vi "DB_EscribeTablaEventos.vi"(8 "error in (no error)":errorcluster, 11 "DESCRIPCION":string) -> (0 "error out":errorcluster)   [LabVIEW 2018]
uses:
  <vilib>/addons/database/Connection.llb/DB Tools Open Connec (Path).vi
  <vilib>/addons/database/Connection.llb/Conn Execute.vi
  <vilib>/addons/database/Recordset.llb/Rec Destroy - Connection.vi
  <vilib>/addons/database/NI_Database_API.lvlib
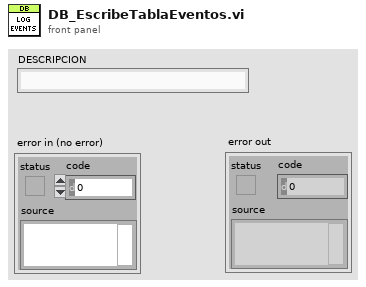
[diagram p1: front panel]
types:
  T1 = typedef "NI_Database_API.lvlib/Conn ObjectReference.ctl" = refnum<k1>
  T2 = typedef "NI_Database_API.lvlib/Rec ObjectReference.ctl" = refnum<k1>
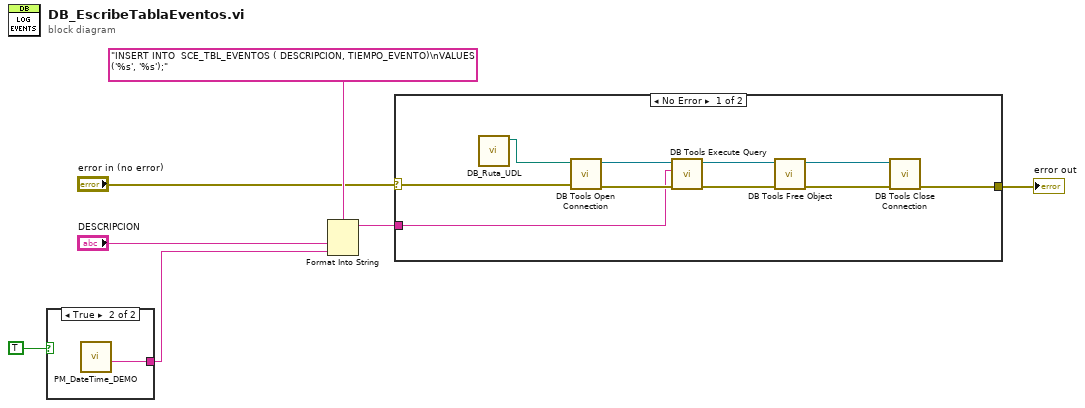
[diagram p0: block diagram]
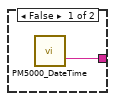
[diagram p2: hidden frame]
diagram:
  n1 = case shown="True" TRUE {
    tunnel: [w8 w9] -> w1
    frame False {
      n2 = call "PM5000_DateTime.vi"() -> ("TIEMPO_MEDICION"=w8:string)  [unwired: 8 in, 3 out]
    }
    frame True {
      n3 = call "PM_DateTime_DEMO.vi"() -> ("TIEMPO_MEDICION"=w9:string)  [unwired: 10 in, 1 out]
    }
  }
  n4 = Format Into String(format string="INSERT INTO  SCE_TBL_EVENTOS ( DESCRIPCION, TIEMPO_EVENTO)\nVALUES ('%s', '%s');" ("SQL"), "DESCRIPCION", w1) -> (resulting string=w7:string)  [unwired: 2 in, 1 out]
  n5 = case shown="No Error" "error in (no error)" {
    selector: "error in (no error)" -> [w12 w20]
    tunnel: w7 -> [w16 _]
    tunnel: [w13 w20] -> w5
    frame No Error {
      n6 = call "DB_Ruta_UDL.vi"() -> ("UDL ruta"=w11:path)  [unwired: 11 in]
      n7 = call-poly <vilib>:"DB Tools Open Connection.vi"("error in (no error)"=w12, "connection information"=w11) -> ("error out"=w19:errorcluster, "connection reference"=w17:T1)  [unwired: 6 in]
      n8 = call-poly <vilib>:"DB Tools Execute Query.vi"("error in (no error)"=w19, "SQL query"=w16, "connection reference"=w17) -> ("error out"=w18:errorcluster, "recordset reference"=w14:T2)  [unwired: 5 in]
      n9 = call-poly <vilib>:"DB Tools Free Object.vi"("error in (no error)"=w18, "recordset reference"=w14) -> ("error out"=w15:errorcluster, "connection reference"=w10:T1)  [unwired: 8 in]
      n10 = call <vilib>:"DB Tools Close Connection.vi"("error in (no error)"=w15, "connection reference"=w10) -> ("error out"=w13:errorcluster)  [unwired: 5 in]
    }
    frame Error {
    }
  }
  "error out" <- w5
